vi "Rauschen RMS.vi"(11 "Eingang":sgl[](array[numeric])=[1.74, 1.82, 1.58, 1.51, 1.45, 2.0, 1.49, 1.72, 1.64, 1.19]) -> (3 "RMS":sgl)   [LabVIEW 2020, in "EPA 1065.lvlib" / "ARN Test 1065-305.lvlib"]
uses:
  ARN Test 1065-305.lvlib
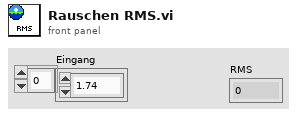
[diagram p1: front panel]
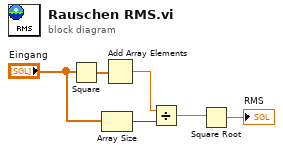
[diagram p0: block diagram]
diagram:
  n1 = Square(x="Eingang") -> (x^2=w2:sgl[])
  n2 = Array Size(array="Eingang") -> (size(s)=w4:i32)
  n3 = Add Array Elements(numeric array=w2) -> (sum=w3:sgl)
  n4 = Divide(x=w3, y=w4) -> (x/y=w5:sgl)
  n5 = Square Root(x=w5) -> (sqrt(x)=→"RMS":sgl)
